vi "Obtain Queues.vi"(8 "error in (no error)":errorcluster) -> (0 "error out":errorcluster, 1 "Q3":refnum<queue>, 2 "Q1":refnum<queue>, 3 "Q2 Cluster":T1)   [LabVIEW 2014]
doc: "<B>Copyright</B>: (c) Ehsan Peymani 2015. All rights reserved.\n\nThis subVI obtains queues that are used for this application and initializes them."
uses:
  TypeDef/Q1 Message.ctl
  Data logger Array Enqueue Function.vi
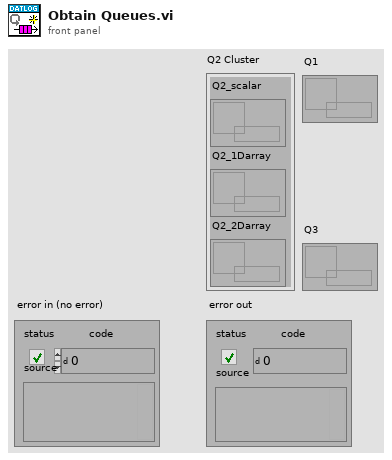
[diagram p1: front panel]
types:
  T1 = cluster{"Q2_scalar":refnum<queue>, "Q2_1Darray":refnum<queue>, "Q2_2Darray":refnum<queue>}
  T2 = typedef "Q1 Message.ctl" = cluster{"state":enum16{"initialize 1", "initialize 2", "initialize 3", "initialize 4", "initialize 5", "initialize 6", "initialize 7", "initialize 8", "initialize 9", "Idle", "Preparation 1", "Preparation 2", "Preparation 3", "Preparation 4", "Record", "Stop recording", "Exit", "Defrag", "View", "Create Database", "Update folder setting", "Update Preference", "Update TDMS properties", "CSV Delimiter", "DB Type", "Hidden Processes", "Replace Database", "Logged File Viewer", "Defrag Prompt File", "View Prompt File", "Save to config file", "Open from config file"}, "data":variant}
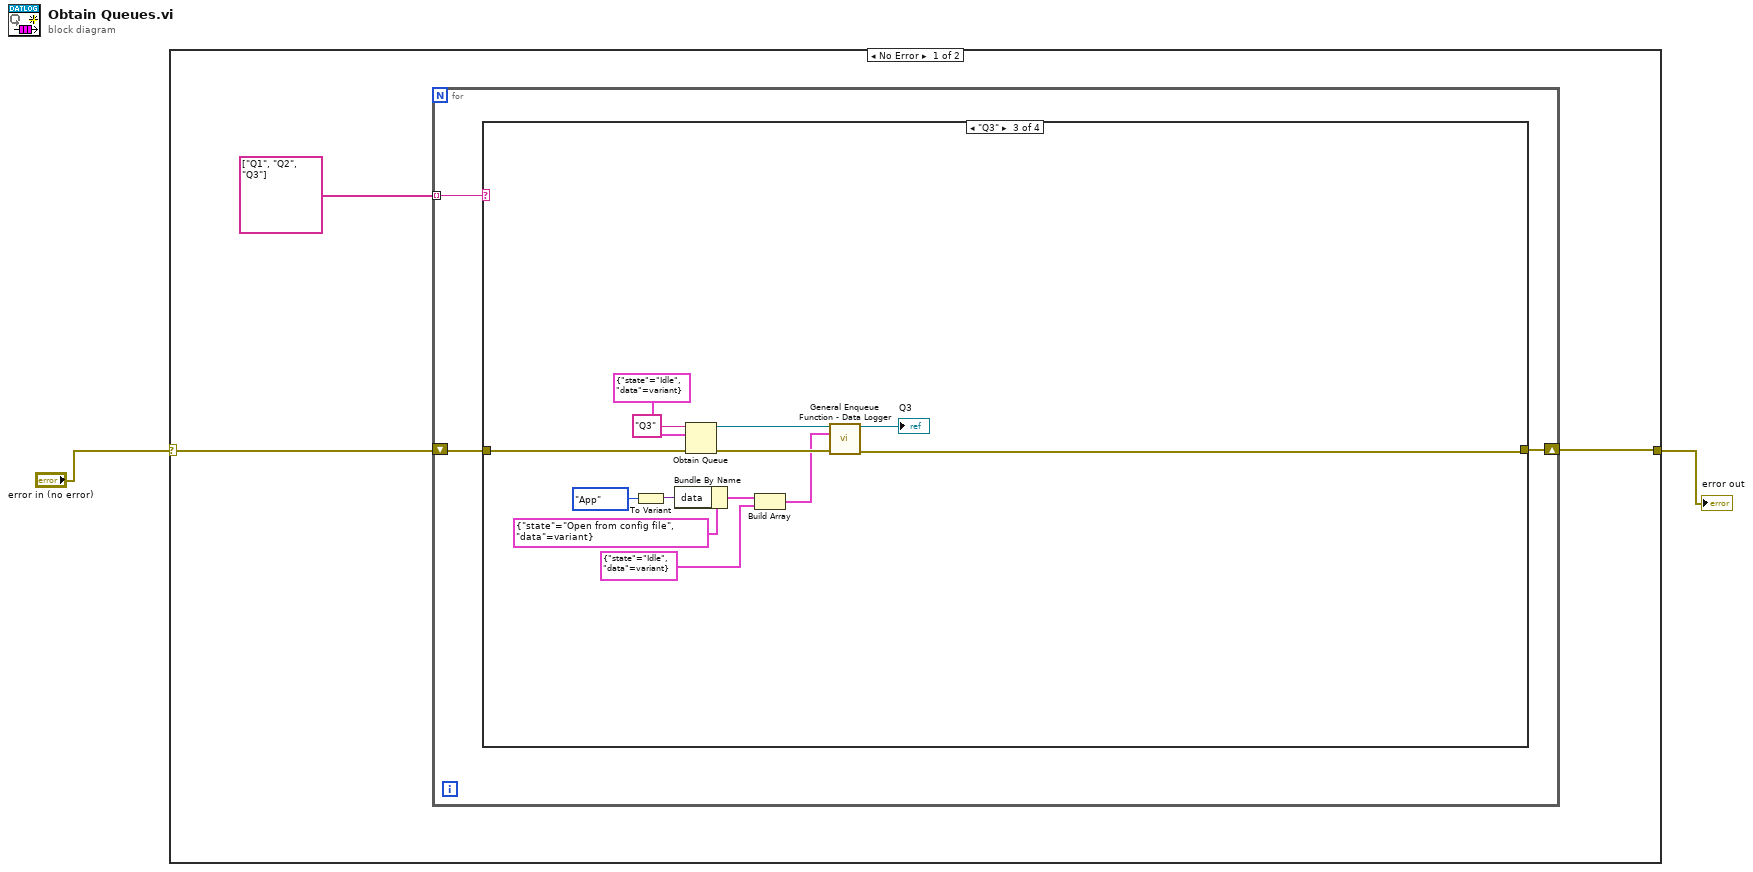
[diagram p0: block diagram]
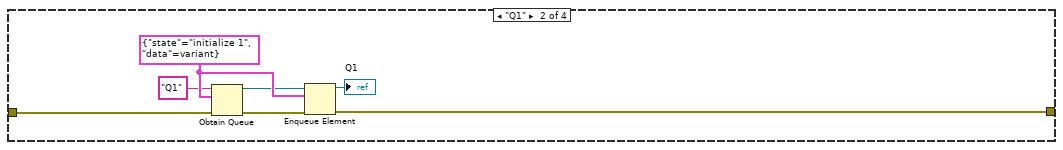
[diagram p3: hidden frame]
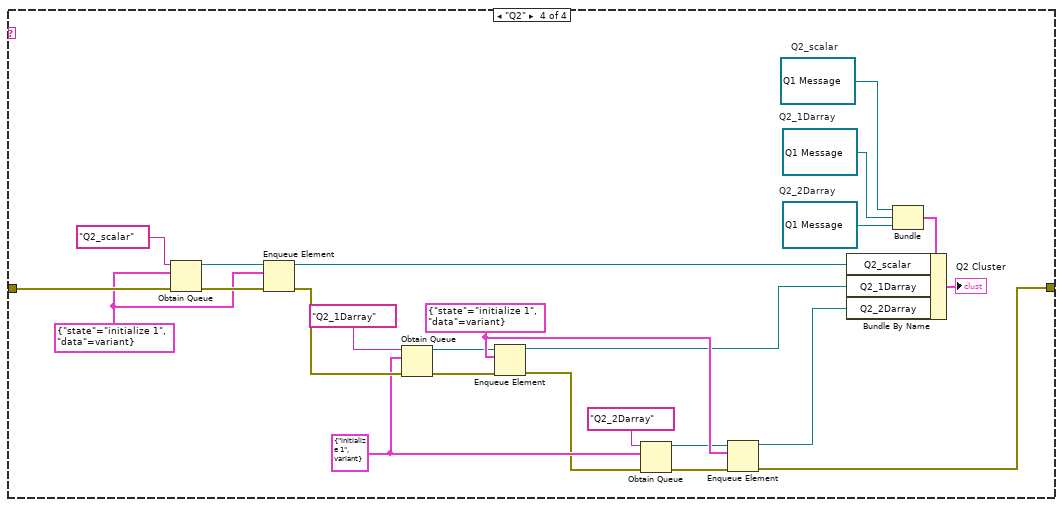
[diagram p4: hidden frame]
diagram:
  n1 = case shown="No Error" "error in (no error)" {
    selector: "error in (no error)" -> [w4 w54]
    tunnel: [w3 w54] -> w1
    frame No Error {
      n2 = for {
        tunnel: string[] ["Q1", "Q2", "Q3"] -> [w8] mode=indexing
        shift-right: [w6] -> w3
        shift-left: w4 -> [w7]
        n3 = case shown="\"Q3\"" w8 {
          tunnel: w7 -> [w9 w12 w27 w37]
          tunnel: [w9 w11 w23 w30] -> w6
          frame "do nothing", Default {
          }
          frame "Q1" {
            w16 = T2 {"state"=enum."initialize 1", "data"=variant} ("Q1 Message")
            n4 = Obtain Queue(name (unnamed)="Q1", element data type=w16, error in (no error)=w12) -> (queue out=w14:refnum<queue>, error out=w15:errorcluster)  [unwired: 2 in, 1 out]
            n5 = Enqueue Element(queue=w14, element=w16, error in (no error)=w15) -> (queue out=→"Q1":refnum<queue>, error out=w11:errorcluster)  [unwired: 1 in, 1 out]
          }
          frame "Q3" {
            n6 = To Variant(anything=enum16{"App", "User"}."App") -> (Variant=w20:variant)
            n7 = Bundle By Name(cluster=T2 {"state"=enum."Open from config file", "data"=variant} ("Q1 Message"), "data"=w20) -> (w22:T2)
            n8 = Obtain Queue(name (unnamed)="Q3", element data type=T2 {"state"=enum."Idle", "data"=variant} ("Q1 Message"), error in (no error)=w27) -> (queue out=w26:refnum<queue>, error out=w24:errorcluster)  [unwired: 2 in, 1 out]
            n9 = Build Array(w22, T2 {"state"=enum."Idle", "data"=variant} ("Q1 Message")) -> (w17:T2[])
            n10 = call-poly "General Enqueue Function - Data Logger.vi"("QRef in"=w26, "Array of Messages"=w17, "Error in"=w24) -> ("QRef out"=→"Q3":refnum<queue>, "Error out"=w23:errorcluster)  [unwired: 11 in]
          }
          frame "Q2" {
            w36 = T2 {"state"=enum."initialize 1", "data"=variant} ("Q1 Message")
            w38 = refnum<queue> refnum  # Q2_2Darray
            w52 = refnum<queue> refnum  # Q2_1Darray
            w53 = refnum<queue> refnum  # Q2_scalar
            w46 = T2 {"state"=enum."initialize 1", "data"=variant} ("Q1 Message")
            w47 = T2 {"state"=enum."initialize 1", "data"=variant} ("Q1 Message")
            n11 = Obtain Queue(name (unnamed)="Q2_scalar", element data type=w36, error in (no error)=w37) -> (queue out=w49:refnum<queue>, error out=w50:errorcluster)  [unwired: 2 in, 1 out]
            n12 = Enqueue Element(queue=w49, element=w36, error in (no error)=w50) -> (queue out=w34:refnum<queue>, error out=w51:errorcluster)  [unwired: 1 in, 1 out]
            n13 = Obtain Queue(name (unnamed)="Q2_1Darray", element data type=w46, error in (no error)=w51) -> (queue out=w40:refnum<queue>, error out=w39:errorcluster)  [unwired: 2 in, 1 out]
            n14 = Enqueue Element(queue=w40, element=w47, error in (no error)=w39) -> (queue out=w33:refnum<queue>, error out=w45:errorcluster)  [unwired: 1 in, 1 out]
            n15 = Obtain Queue(name (unnamed)="Q2_2Darray", element data type=w46, error in (no error)=w45) -> (queue out=w43:refnum<queue>, error out=w44:errorcluster)  [unwired: 2 in, 1 out]
            n16 = Enqueue Element(queue=w43, element=w47, error in (no error)=w44) -> (queue out=w32:refnum<queue>, error out=w30:errorcluster)  [unwired: 1 in, 1 out]
            n17 = Bundle("Q2_scalar"=w53, "Q2_1Darray"=w52, "Q2_2Darray"=w38) -> (w35:T1)  [unwired: 1 in]
            n18 = Bundle By Name(cluster=w35, "Q2_scalar"=w34, "Q2_1Darray"=w33, "Q2_2Darray"=w32) -> (→"Q2 Cluster":T1)
          }
        }
      }
    }
    frame Error {
    }
  }
  "error out" <- w1
